vi "Run G-AI Tests CICD.vi"() -> ()   [LabVIEW 2020]
doc: "Wrapper to run all tests and pass result to LabVIEW CLI.\nConnectorpane of this VI cannot be changed."
uses:
  <vilib>/addons/_JKI Toolkits/Caraya/classes/Test Suite/Test Suite.lvclass
  <vilib>/addons/_JKI Toolkits/Caraya/classes/Test Suite/Define Test Suite (Default).vi
  G-AI tests.lvlib
panel:
  out "Exit Code":i32
  in  "Command Line Arguments":string[](array[string])
  out "Output":string
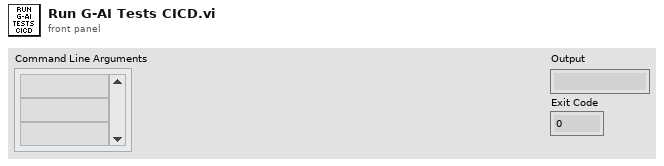
[diagram p1: front panel]
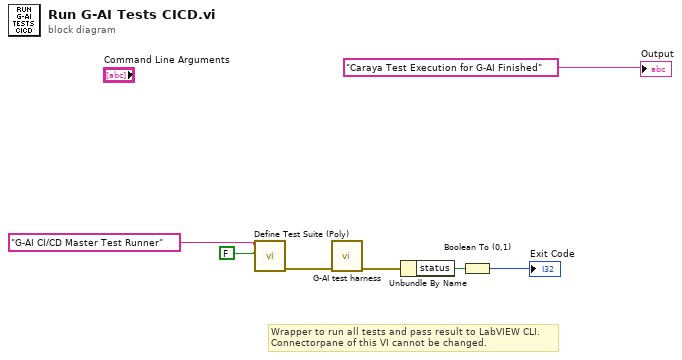
[diagram p0: block diagram]
diagram:
  # "Wrapper to run all tests and pass result to LabVIEW CLI.\nConnectorpane of this VI cannot be changed."
  n1 = call-poly <vilib>:"Define Test Suite (Poly).vi"("Interactive"=FALSE, "Label (VI Title)"="G-AI CI/CD Master Test Runner") -> ("error out"=w2:errorcluster)  [unwired: 7 in, 2 out]
  n2 = call "G-AI test harness.vi"("error in"=w2) -> ("error out"=w1:errorcluster)  [unwired: 10 in]
  n3 = Unbundle By Name(w1) -> ("status"=w5:bool)
  n4 = Boolean To (0,1)(Boolean=w5) -> (0, 1=→"Exit Code":i16)
  "Output" <- "Caraya Test Execution for G-AI Finished" ("Output")
